vi "Load Config.vi"(8 "error in (no error)":errorcluster, 11 "Config-YAML in":refnum<class "Config-YAML.lvclass">) -> (0 "error out":errorcluster, 2 "Elements":T1[](array[typedef]), 3 "Config-YAML out":refnum<class "Config-YAML.lvclass">)   [LabVIEW 2020, in "CDM-Config.lvlib" / "Config-YAML.lvclass"]
uses:
  Config-YAML.lvclass
  Config Element.ctl
  Meta Data.ctl
  Value Type.ctl
  CDM-Config.lvlib
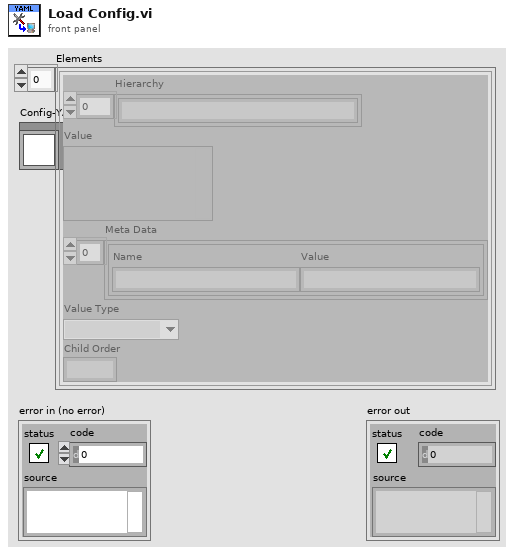
[diagram p1: front panel]
types:
  T1 = typedef "CDM-Config.lvlib/Config Element.ctl" = cluster{"Hierarchy":string[], "Value":variant, "Meta Data":T2[], "Value Type":T3, "Child Order":i32}
  T2 = typedef "CDM-Config.lvlib/Meta Data.ctl" = cluster{"Name":string, "Value":string}
  T3 = typedef "CDM-Config.lvlib/Value Type.ctl" = enum16{"String", "Number", "Bool", "Object", "Array"}
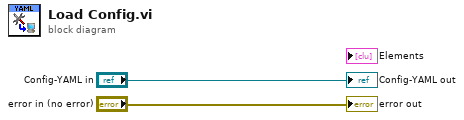
[diagram p0: block diagram]
diagram:
  "error out" <- "error in (no error)"
  "Config-YAML out" <- "Config-YAML in"
